vi "Zero Crossing (DBL Array).vi"(2 "initialize":bool, 3 "direction":enum16{"either", "minus-plus", "plus-minus"}(ring), 5 "Input Points":dbl[](array[numeric]) format="%.2f") -> (1 "Crossings":bool[](array[boolean]))   [LabVIEW 2017, in "NI_AdvCtrl_nonlinear.lvlib"]
doc: "LabVIEW no longer supports this VI. You can obtain similar functionality by installing the LabVIEW Simulation Module.\n\nDetects zero crossings of the input signal. The user can choose from three different detectors, either, minus-plus, and plus-minus."
uses:
  <vilib>/addons/control/advanced/NI_AdvCtrl_nonlinear.lvlib
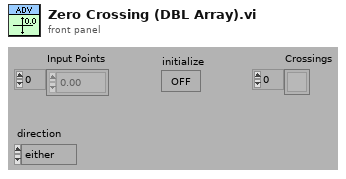
[diagram p1: front panel]
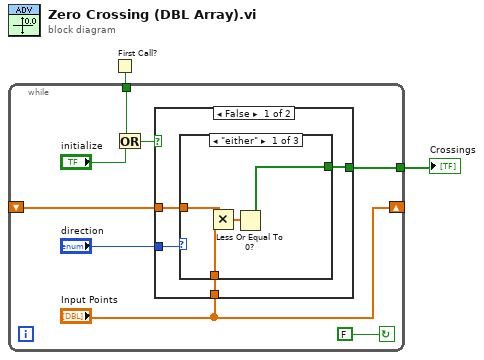
[diagram p0: block diagram]
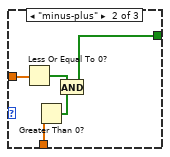
[diagram p2: hidden frame]
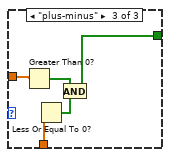
[diagram p3: hidden frame]
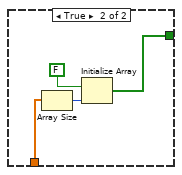
[diagram p4: hidden frame]
diagram:
  n1 = First Call?() -> (First Call?: T/F=w2:bool)
  n2 = while {
    tunnel: w2 -> [w5]
    tunnel: [w10] -> w1
    shift-left: _ -> [w8]
    shift-right: ["Input Points"] -> _
    stop <- FALSE continue-if-true
    n3 = Or(x=w5, y="initialize") -> (x .or. y?=w6:bool)
    n4 = case shown="False" w6 {
      tunnel: [w11 w29] -> w10
      tunnel: "direction" -> [w14 _]
      tunnel: w8 -> [w13 _]
      tunnel: "Input Points" -> [w12 w31]
      frame False {
        n5 = case shown="\"either\"" w14 {
          tunnel: w13 -> [w18 w23 w28]
          tunnel: w12 -> [w17 w22 w24]
          tunnel: [w15 w19 w25] -> w11
          frame "either" {
            n6 = Multiply(x=w18, y=w17) -> (x*y=w16:dbl[])
            n7 = Less Or Equal To 0?(x=w16) -> (x <= 0?=w15:bool[])
          }
          frame "minus-plus" {
            n8 = Less Or Equal To 0?(x=w23) -> (x <= 0?=w21:bool[])
            n9 = Greater Than 0?(x=w22) -> (x > 0?=w20:bool[])
            n10 = And(x=w21, y=w20) -> (x .and. y?=w19:bool[])
          }
          frame "plus-minus" {
            n11 = Greater Than 0?(x=w28) -> (x > 0?=w27:bool[])
            n12 = Less Or Equal To 0?(x=w24) -> (x <= 0?=w26:bool[])
            n13 = And(x=w27, y=w26) -> (x .and. y?=w25:bool[])
          }
        }
      }
      frame True {
        n14 = Array Size(array=w31) -> (size(s)=w32:i32)
        n15 = Initialize Array(FALSE, w32) -> (w29:bool[])
      }
    }
  }
  "Crossings" <- w1
